vi "Nelder-Mead_alignment-max.vi"() -> (3 "Optimized Location":dbl[](array[numeric]), 10 "yStart":dbl=123.0 format="%#_13g", 11 "xStart":dbl=264.0 format="%#_13g")   [LabVIEW 2024]
uses:
  <vilib>/numeric/Random Number (Range) DBL.vi
  0b4b40c4-ef97-49a3-bff4-9c7e9883bc37.vi
  5b59031f-b1ff-41af-80a7-e72a33ebffa1.vi
  <vilib>/Array/Sort 2D Array - Pop Stack.vi
  <vilib>/Array/Sort 2D Array - Push Stack.vi
  0b4b40c4-ef97-49a3-bff4-9c7e9883bc37.vi/269d4b3b-47f5-49e3-8884-44851e4dd9d5.vi
  0b4b40c4-ef97-49a3-bff4-9c7e9883bc37.vi/6d99389c-673d-4efb-bf33-19b32bcf4cf8.vi
  5b59031f-b1ff-41af-80a7-e72a33ebffa1.vi/269d4b3b-47f5-49e3-8884-44851e4dd9d5.vi
  5b59031f-b1ff-41af-80a7-e72a33ebffa1.vi/6d99389c-673d-4efb-bf33-19b32bcf4cf8.vi
  <vilib>/Analysis/NI_AALBase.lvlib
panel:
  out "model-mode":bool
  out "elapsed time (s)":dbl
  out "n":i32(slide) scale=0.0..1000.0
  out "GrAsc - avgs":dbl[][](array[numeric])
  out "NM - avgs":dbl[][](array[numeric])
  in  "nTrials":i32=1000
  out "std dev of simplex values 2":dbl
  out "simplex leg lengths 2":dbl[](array[numeric])
  out "iterations timeout 2":bool
  out "simplex converge 2":bool
  out "value converge 2":bool
  out "Starting Points":dbl[][][](array[numeric])
  in  "k":dbl=50.0
  out "GrAsc res":dbl[](array[numeric])
  out "x_c":dbl[](array[numeric])
  out "x_e":dbl[](array[numeric])
  out "x_r":dbl[](array[numeric])
  out "x_o":dbl[](array[numeric])
  out "iterations timeout":bool
  out "simplex converge":bool
  out "value converge":bool
  out "simplex leg lengths":dbl[](array[numeric])
  out "std dev of simplex values":dbl
  in  "stop":bool
  # "Avg"
  # "Std Dev"
  # "X"
  # "Y"
  # "Value"
  # "n Trials"
  # "Failures"
  # "Avg"
  # "Std Dev"
  # "X"
  # "Y"
  # "Value"
  # "n Trials"
  # "Failures"
  # "centroid"
  # "reflection point"
  # "expansion point"
  # "contraction point"
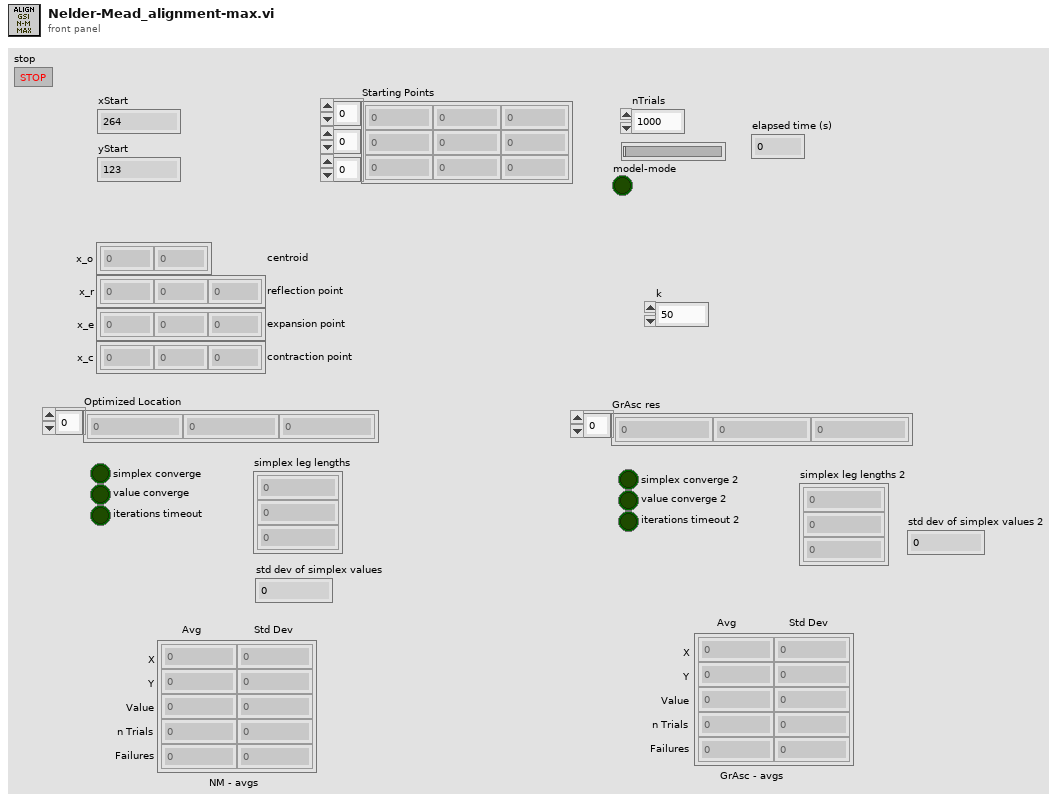
[diagram p1: front panel]
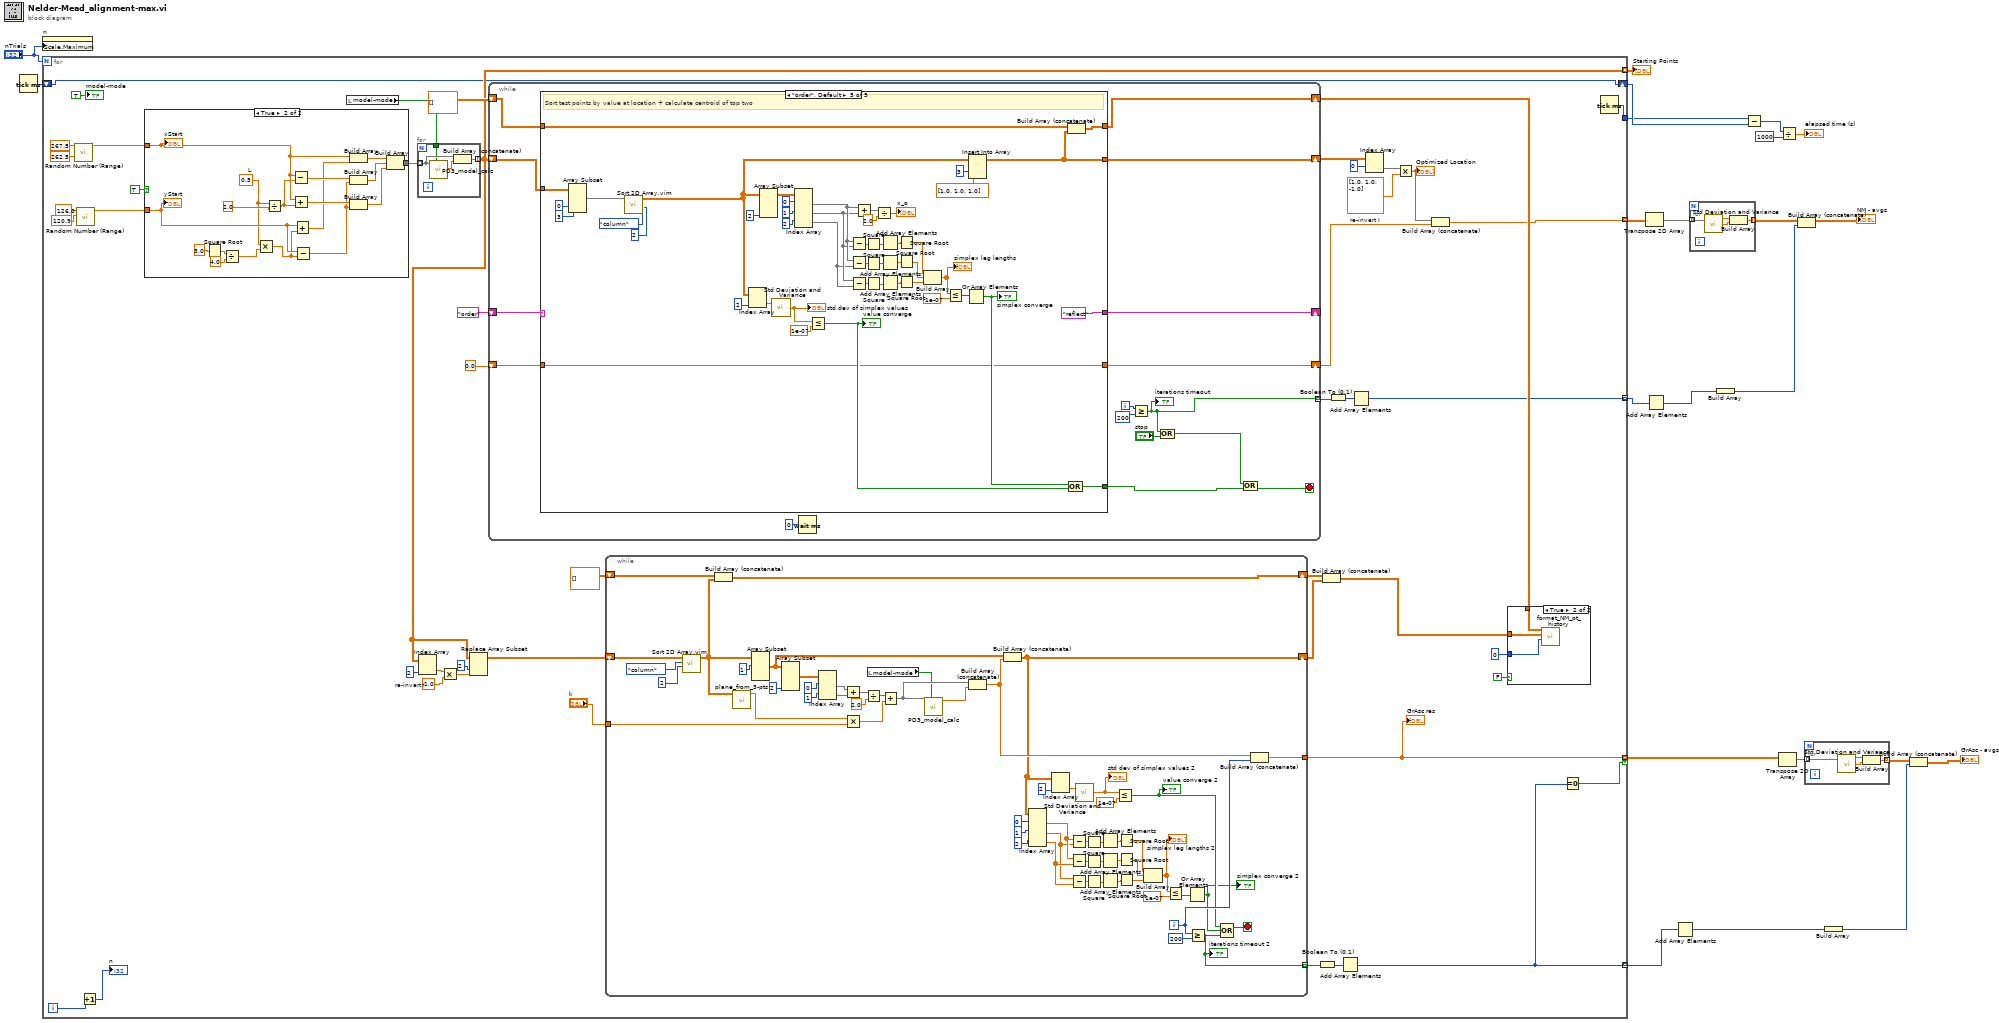
[diagram p0: block diagram]
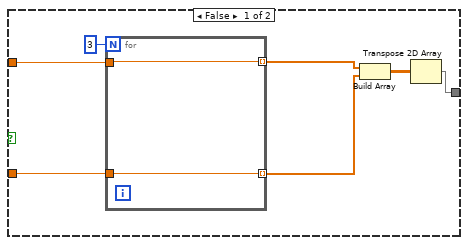
[diagram p3: hidden frame]
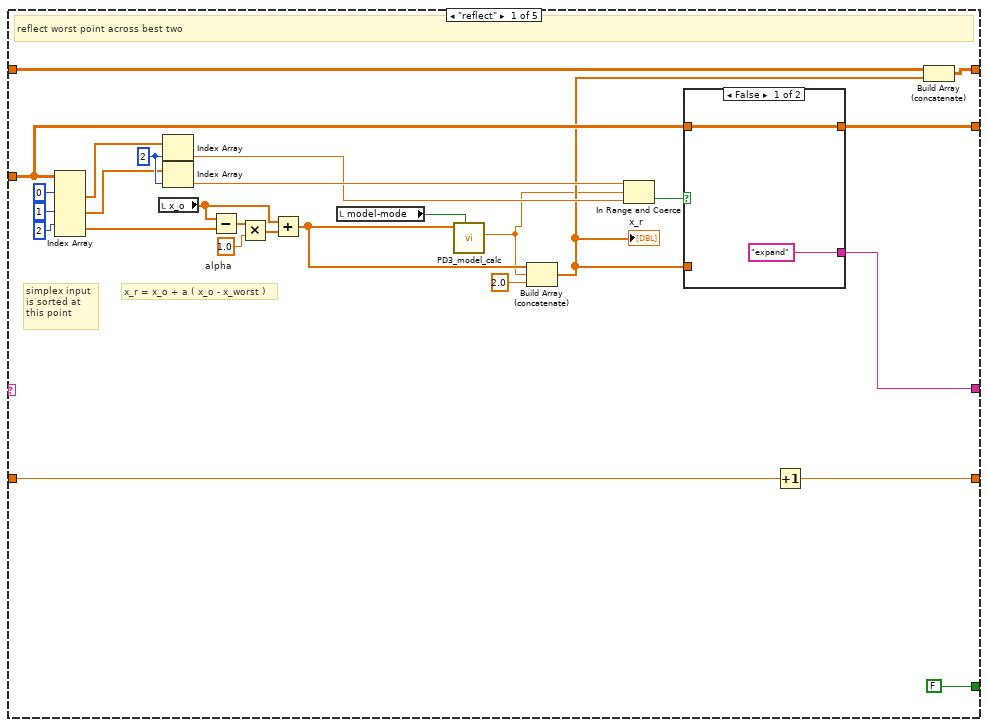
[diagram p4: hidden frame]
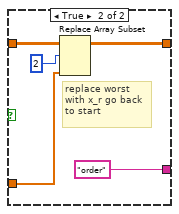
[diagram p5: hidden frame]
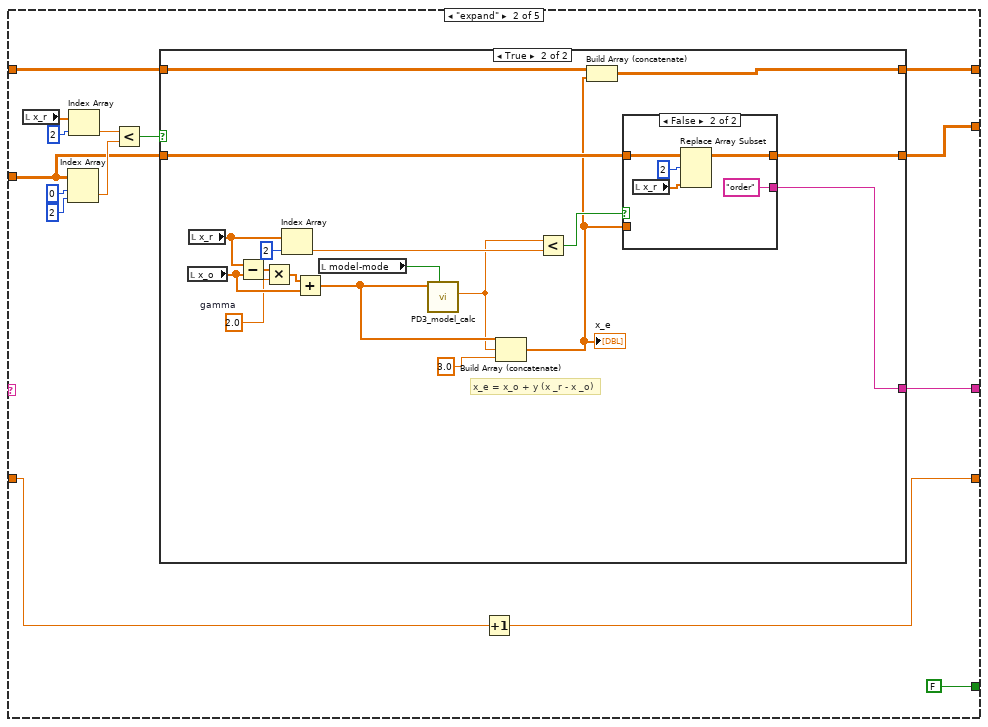
[diagram p6: hidden frame]
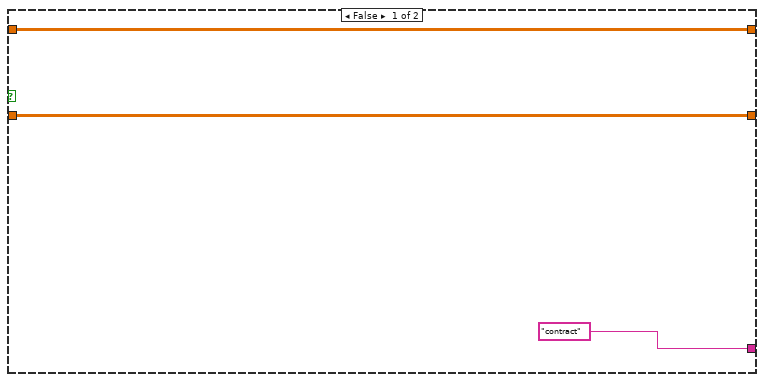
[diagram p7: hidden frame]
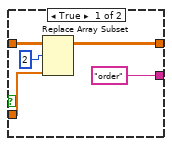
[diagram p8: hidden frame]
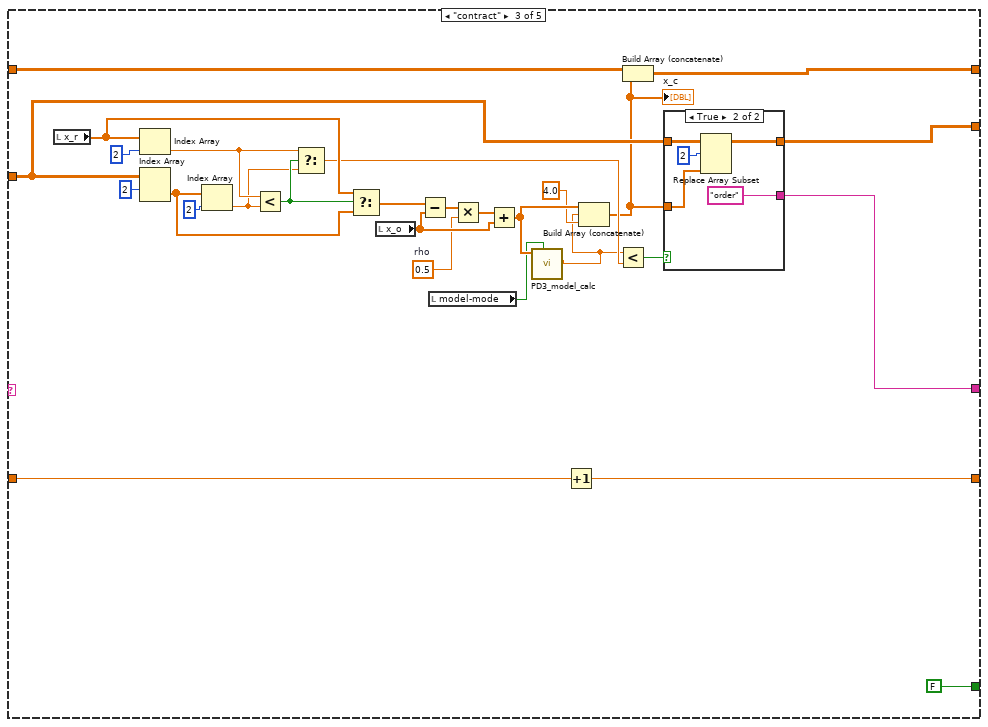
[diagram p9: hidden frame]
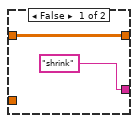
[diagram p10: hidden frame]
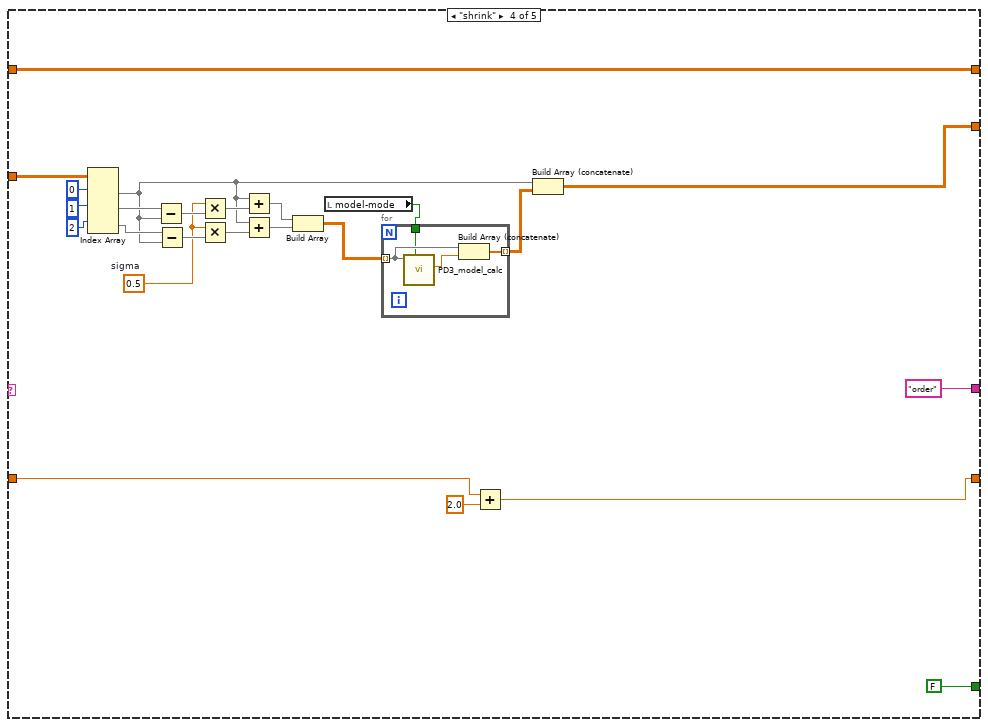
[diagram p11: hidden frame]
diagram:
  n1 = Tick Count (ms)() -> (millisecond timer value=w4:u32)
  n2 = property on="n" class="Slide (strict)"("Scale.Maximum"="nTrials") -> ()  [unwired: 2 in, 2 out]
  n3 = for {
    N: "nTrials" -> [_]
    tunnel: [w42] -> w21 mode=indexing
    tunnel: [w40] -> w20 mode=indexing
    tunnel: [w37] -> w15 mode=indexing if=w34
    tunnel: [w33] -> w14 mode=indexing
    tunnel: [w30] -> w10 mode=indexing
    shift-right: [w26] -> w3
    shift-left: w4 -> [w26]
    tunnel: [w25] -> w1
    i -> [w29]
    w57 = -1.0  # re-invert I
    w64 = dbl[] [1.0, 1.0, -1.0]  # re-invert I
    n4 = call-poly <vilib>:"Random Number (Range).vi"("lower bound (0)"=262.5, "upper bound (100)"=267.5) -> ("number"=w48:dbl)  [unwired: 9 in]
    n5 = call-poly <vilib>:"Random Number (Range).vi"("lower bound (0)"=120.9 ("upper bound (100)"), "upper bound (100)"=126.0 ("lower bound (0)")) -> ("number"=w47:dbl)  [unwired: 9 in]
    n6 = Increment(x=w29) -> (x+1=→"n":i32)
    n7 = case shown="True" TRUE {
      tunnel: [w73 w96] -> w52
      tunnel: w48 -> [w78 w88]
      tunnel: w47 -> [w77 w87]
      frame False {
        n8 = for {
          N: 3 -> [_]
          tunnel: w78 -> [w81]
          tunnel: [w81] -> w76 mode=indexing
          tunnel: w77 -> [w80]
          tunnel: [w80] -> w74 mode=indexing
        }
        n9 = Build Array(w76, w74) -> (w75:dbl[][])
        n10 = Transpose 2D Array(2D array=w75) -> (transposed array=w73:dbl[][])
      }
      frame True {
        w82 = 0.5  # L
        n11 = Square Root(x=3.0) -> (sqrt(x)=w95:dbl)
        n12 = Divide(x=w95, y=4.0) -> (x/y=w84:dbl)
        n13 = Multiply(x=w82, y=w84) -> (x*y=w83:dbl)
        n14 = Divide(x=w82, y=2.0) -> (x/y=w85:dbl)
        n15 = Subtract(x=w88, y=w85) -> (x-y=w92:dbl)
        n16 = Add(x=w88, y=w85) -> (x+y=w91:dbl)
        n17 = Add(x=w87, y=w83) -> (x+y=w90:dbl)
        n18 = Subtract(x=w87, y=w83) -> (x-y=w89:dbl)
        n19 = Build Array(w88, w90) -> (w97:dbl[])
        n20 = Build Array(w92, w89) -> (w98:dbl[])
        n21 = Build Array(w91, w89) -> (w99:dbl[])
        n22 = Build Array(w97, w98, w99) -> (w96:dbl[][])
        "xStart" <- w88
        "yStart" <- w87
      }
    }
    n23 = local read "model-mode"() -> (w23:bool)
    n24 = for {
      tunnel: w52 -> [w159] mode=indexing
      tunnel: [w160] -> w42 mode=indexing
      tunnel: w23 -> [w157]
      n25 = call "PD3_model_calc.vi"("mode"=w157, "pos_in"=w159) -> ("-I_out"=w158:dbl)  [unwired: 8 in, 1 out]
      n26 = Build Array (concatenate)(w159, w158) -> (w160:dbl[])
    }
    n27 = Index Array(array=w42, index (col)=2 ("disabled index (col)")) -> (element=w55:dbl[])  [unwired: 1 in]
    n28 = Multiply(x=w55, y=w57) -> (x*y=w53:dbl[])
    n29 = Replace Array Subset(array=w42, new element=w53, index (col)=2 ("disabled index (col)")) -> (w51:dbl[][])  [unwired: 1 in]
    n30 = while {
      shift-right: [w174] -> w69
      shift-left: w42 -> [w172]
      shift-right: [w175] -> _
      shift-left: "order" -> [w176]
      shift-right: [w170] -> w63
      shift-left: dbl[][] [] -> [w171]
      shift-right: [w164] -> w38
      shift-left: 0.0 -> [w165]
      tunnel: [w163] -> w31 mode=indexing
      i -> [w166]
      stop <- w162 stop-if-true
      n31 = case shown="\"order\", Default" w176 {
        tunnel: w172 -> [w188 w218 w270 w314 w358]
        tunnel: [FALSE FALSE FALSE FALSE w334] -> w168
        tunnel: [w187 w217 w271 w303 w323] -> w174
        tunnel: [w189 w216 w272 "order" "reflect"] -> w175
        tunnel: w171 -> [w185 w214 w266 w301 w322]
        tunnel: [w184 w213 w264 w301 w328] -> w170
        tunnel: w165 -> [w180 w212 w260 w295 w320]
        tunnel: [w179 w211 w259 w294 w320] -> w164
        frame "reflect" {
          w181 = 1.0  # alpha
          w197 = 2 ("index")
          # "simplex input\nis sorted at\nthis point"
          # "x_r = x_o + a ( x_o - x_worst )"
          # "reflect worst point across best two"
          n32 = Index Array(array=w188, index (row) #1=0 ("index (row)"), index (row) #2=1 ("index (row)"), index (row) #3=2 ("index (row)")) -> (element #1=w196:dbl[], element #2=w195:dbl[], element #3=w198:dbl[])  [unwired: 3 in]
          n33 = local read "x_o"() -> (w190:dbl[])
          n34 = Index Array(array=w196, index=w197) -> (element=w193:dbl)
          n35 = Index Array(array=w195, index=w197) -> (element=w194:dbl)
          n36 = Subtract(x=w190, y=w198) -> (x-y=w202:dbl[])
          n37 = Multiply(x=w202, y=w181) -> (x*y=w201:dbl[])
          n38 = Add(x=w190, y=w201) -> (x+y=w191:dbl[])
          n39 = local read "model-mode"() -> (w177:bool)
          n40 = call "PD3_model_calc.vi"("mode"=w177, "pos_in"=w191) -> ("-I_out"=w178:dbl)  [unwired: 8 in, 1 out]
          n41 = Build Array (concatenate)(w191, w178, 2.0) -> (w183:dbl[])
          "x_r" <- w183
          n42 = In Range and Coerce(upper limit=w194, x=w178, lower limit=w193) -> (In Range?=w192:bool)  [unwired: 1 out]
          n43 = case shown="False" w192 {
            tunnel: ["expand" "order"] -> w189
            tunnel: w188 -> [w204 w210]
            tunnel: [w204 w207] -> w187
            tunnel: w183 -> [_ w208]
            frame False {
            }
            frame True {
              # "replace worst \nwith x_r go back\nto start"
              n44 = Replace Array Subset(array=w210, new element=w208, index (row)=2) -> (w207:dbl[][])  [unwired: 1 in]
            }
          }
          n45 = Increment(x=w180) -> (x+1=w179:dbl)
          n46 = Build Array (concatenate)(w185, w183) -> (w184:dbl[][])
        }
        frame "expand" {
          n47 = local read "x_r"() -> (w223:dbl[])
          n48 = Index Array(array=w218, index (row)=0, index (col)=2 ("disabled index (col)")) -> (element=w221:dbl)
          n49 = Index Array(array=w223, index=2) -> (element=w220:dbl)
          n50 = Less?(x=w220, y=w221) -> (x < y?=w219:bool)
          n51 = case shown="True" w219 {
            tunnel: w218 -> [w228 w239]
            tunnel: [w228 w237] -> w217
            tunnel: ["contract" w236] -> w216
            tunnel: w214 -> [w226 w235]
            tunnel: [w226 w234] -> w213
            frame False {
            }
            frame True {
              w231 = 2.0  # gamma
              # "x_e = x_o + y (x _r - x _o)"
              n52 = local read "x_o"() -> (w244:dbl[])
              n53 = local read "x_r"() -> (w243:dbl[])
              n54 = Subtract(x=w243, y=w244) -> (x-y=w246:dbl[])
              n55 = Multiply(x=w246, y=w231) -> (x*y=w245:dbl[])
              n56 = Index Array(array=w243, index=2) -> (element=w241:dbl)
              n57 = Add(x=w245, y=w244) -> (x+y=w238:dbl[])
              n58 = local read "model-mode"() -> (w229:bool)
              n59 = call "PD3_model_calc.vi"("mode"=w229, "pos_in"=w238) -> ("-I_out"=w230:dbl)  [unwired: 8 in, 1 out]
              n60 = Build Array (concatenate)(w238, w230, 3.0) -> (w233:dbl[])
              "x_e" <- w233
              n61 = Less?(x=w230, y=w241) -> (x < y?=w240:bool)
              n62 = Build Array (concatenate)(w235, w233) -> (w234:dbl[][])
              n63 = case shown="False" w240 {
                tunnel: w239 -> [w250 w255]
                tunnel: w233 -> [w249 _]
                tunnel: [w248 w254] -> w237
                tunnel: ["order" "order"] -> w236
                frame True {
                  n64 = Replace Array Subset(array=w250, new element=w249, index (row)=2) -> (w248:dbl[][])  [unwired: 1 in]
                }
                frame False {
                  n65 = local read "x_r"() -> (w252:dbl[])
                  n66 = Replace Array Subset(array=w255, new element=w252, index (row)=2) -> (w254:dbl[][])  [unwired: 1 in]
                }
              }
            }
          }
          n67 = Increment(x=w212) -> (x+1=w211:dbl)
        }
        frame "contract" {
          w261 = 0.5  # rho
          n68 = local read "x_r"() -> (w281:dbl[])
          n69 = Index Array(array=w281, index=2) -> (element=w276:dbl)
          n70 = Index Array(array=w270, index (row)=2) -> (element=w280:dbl[])  [unwired: 1 in]
          n71 = Index Array(array=w280, index=2) -> (element=w275:dbl)
          n72 = Less?(x=w276, y=w275) -> (x < y?=w277:bool)
          n73 = Select(t=w276, s=w277, f=w275) -> (s? t:f=w274:dbl)
          n74 = Select(t=w281, s=w277, f=w280) -> (s? t:f=w279:dbl[])
          n75 = local read "x_o"() -> (w268:dbl[])
          n76 = Subtract(x=w279, y=w268) -> (x-y=w278:dbl[])
          n77 = local read "model-mode"() -> (w257:bool)
          n78 = Multiply(x=w278, y=w261) -> (x*y=w269:dbl[])
          n79 = Add(x=w269, y=w268) -> (x+y=w265:dbl[])
          n80 = call "PD3_model_calc.vi"("mode"=w257, "pos_in"=w265) -> ("-I_out"=w258:dbl)  [unwired: 8 in, 1 out]
          n81 = Increment(x=w260) -> (x+1=w259:dbl)
          n82 = Build Array (concatenate)(w265, w258, 4.0 ("array")) -> (w263:dbl[])
          "x_c" <- w263
          n83 = Less?(x=w258, y=w274) -> (x < y?=w273:bool)
          n84 = Build Array (concatenate)(w266, w263) -> (w264:dbl[][])
          n85 = case shown="True" w273 {
            tunnel: ["shrink" "order"] -> w272
            tunnel: [w285 w287] -> w271
            tunnel: w270 -> [w285 w289]
            tunnel: w263 -> [_ w288]
            frame False {
            }
            frame True {
              n86 = Replace Array Subset(array=w289, new element=w288, index (row)=2) -> (w287:dbl[][])  [unwired: 1 in]
            }
          }
        }
        frame "shrink" {
          w300 = 0.5  # sigma
          n87 = Index Array(array=w314, index (row) #1=0 ("index (row)"), index (row) #2=1 ("index (row)"), index (row) #3=2 ("index (row)")) -> (element #1=w304:dbl[], element #2=w310:dbl[], element #3=w309:dbl[])  [unwired: 3 in]
          n88 = Subtract(x=w310, y=w304) -> (x-y=w307:dbl[])
          n89 = Subtract(x=w309, y=w304) -> (x-y=w308:dbl[])
          n90 = Multiply(x=w300, y=w307) -> (x*y=w306:dbl[])
          n91 = Multiply(x=w300, y=w308) -> (x*y=w305:dbl[])
          n92 = Add(x=w304, y=w306) -> (x+y=w299:dbl[])
          n93 = Add(x=w304, y=w305) -> (x+y=w298:dbl[])
          n94 = Build Array(w299, w298) -> (w297:dbl[][])
          n95 = local read "model-mode"() -> (w292:bool)
          n96 = for {
            tunnel: w297 -> [w318] mode=indexing
            tunnel: [w319] -> w296 mode=indexing
            tunnel: w292 -> [w316]
            n97 = call "PD3_model_calc.vi"("mode"=w316, "pos_in"=w318) -> ("-I_out"=w317:dbl)  [unwired: 8 in, 1 out]
            n98 = Build Array (concatenate)(w318, w317) -> (w319:dbl[])
          }
          n99 = Add(x=w295, y=2.0) -> (x+y=w294:dbl)
          n100 = Build Array (concatenate)(w304, w296) -> (w303:dbl[][])
        }
        frame "order", Default {
          # "Sort test points by value at location + calculate centroid of top two"
          n101 = Array Subset(array=w358, index (col)=0 ("index"), length (col)=3 ("length")) -> (w321:dbl[][])  [unwired: 2 in]
          n102 = call "Sort 2D Array.vim"("index"=2, "dimension to index (column)"=enum16{"column", "row"}."column", "2D array"=w321) -> ("sorted 2D array"=w326:dbl[][])  [unwired: 7 in, 1 out]
          n103 = Index Array(array=w326, index (col)=2 ("index")) -> (element=w352:dbl[])  [unwired: 1 in]
          n104 = Array Subset(array=w326, length (col)=2 ("length")) -> (w351:dbl[][])  [unwired: 3 in]
          n105 = call <vilib>:"Std Deviation and Variance.vi"("X"=w352) -> ("standard deviation"=w327:dbl)  [unwired: 1 in, 2 out]
          "std dev of simplex values" <- w327
          n106 = Index Array(array=w351, index (row) #1=0 ("index (row)"), index (row) #2=1 ("index (row)"), index (row) #3=2 ("index (row)")) -> (element #1=w331:dbl[], element #2=w330:dbl[], element #3=w329:dbl[])  [unwired: 3 in]
          n107 = Less Or Equal?(x=w327, y=1e-07) -> (x <= y?=w333:bool)
          "value converge" <- w333
          n108 = Subtract(x=w331, y=w330) -> (x-y=w349:dbl[])
          n109 = Subtract(x=w331, y=w329) -> (x-y=w341:dbl[])
          n110 = Subtract(x=w330, y=w329) -> (x-y=w344:dbl[])
          n111 = Add(x=w331, y=w330) -> (x+y=w356:dbl[])
          n112 = Square(x=w349) -> (x^2=w348:dbl[])
          n113 = Square(x=w341) -> (x^2=w345:dbl[])
          n114 = Square(x=w344) -> (x^2=w343:dbl[])
          n115 = Divide(x=w356, y=2.0) -> (x/y=→"x_o":dbl[])
          n116 = Add Array Elements(numeric array=w348) -> (sum=w347:dbl)
          n117 = Add Array Elements(numeric array=w345) -> (sum=w346:dbl)
          n118 = Add Array Elements(numeric array=w343) -> (sum=w342:dbl)
          n119 = Square Root(x=w347) -> (sqrt(x)=w338:dbl)
          n120 = Square Root(x=w346) -> (sqrt(x)=w339:dbl)
          n121 = Square Root(x=w342) -> (sqrt(x)=w340:dbl)
          n122 = Build Array(w338, w339, w340) -> (w337:dbl[])
          "simplex leg lengths" <- w337
          n123 = Less Or Equal?(x=w337, y=1e-07) -> (x <= y?=w335:bool[])
          n124 = Or Array Elements(Boolean array=w335) -> (logical OR=w332:bool)
          "simplex converge" <- w332
          n125 = Insert Into Array(array=w326, index (col)=3 ("disabled index (col)"), new element=dbl[] [1.0, 1.0, 1.0] ("new element/subarray")) -> (w323:dbl[][])  [unwired: 1 in]
          n126 = Build Array (concatenate)(w322, w323) -> (w328:dbl[][])
          n127 = Compound Arithmetic op=OR(w332, w333) -> (w334:bool)
        }
      }
      n128 = Wait (ms)(milliseconds to wait=u32 0) -> ()  [unwired: 1 out]
      n129 = Greater Or Equal?(x=w166, y=200) -> (x >= y?=w163:bool)
      "iterations timeout" <- w163
      n130 = Compound Arithmetic op=OR(w163, "stop") -> (w161:bool)
      n131 = Compound Arithmetic op=OR(w161, w168) -> (w162:bool)
    }
    n132 = while {
      tunnel: "k" -> [w134]
      shift-right: [w137] -> w50
      shift-left: dbl[][] [] -> [w156]
      shift-right: [w115] -> w49
      shift-left: w51 -> [w153]
      tunnel: [w129] -> w37
      tunnel: [w102] -> w36 mode=indexing
      i -> [w128]
      stop <- w130 stop-if-true
      n133 = call "Sort 2D Array.vim"("index"=2, "dimension to index (column)"=enum16{"column", "row"}."column", "2D array"=w153) -> ("sorted 2D array"=w136:dbl[][])  [unwired: 7 in, 1 out]
      n134 = Build Array (concatenate)(w156, w136) -> (w137:dbl[][])
      n135 = call "plane_from_3-pts.vi"("Input"=w136) -> ("gradient-out"=w139:dbl[])  [unwired: 9 in, 1 out]
      n136 = Array Subset(array=w136, index (row)=1 ("index")) -> (w143:dbl[][])  [unwired: 3 in]
      n137 = Array Subset(array=w143, length (col)=2 ("length")) -> (w144:dbl[][])  [unwired: 3 in]
      n138 = Index Array(array=w144, index (row) #1=0 ("index (row)"), index (row) #2=1 ("index (row)")) -> (element #1=w149:dbl[], element #2=w148:dbl[])  [unwired: 2 in]
      n139 = Add(x=w149, y=w148) -> (x+y=w147:dbl[])
      n140 = Multiply(x=w139, y=w134) -> (x*y=w140:dbl[])
      n141 = Divide(x=w147, y=2.0) -> (x/y=w142:dbl[])
      n142 = local read "model-mode"() -> (w100:bool)
      n143 = Add(x=w142, y=w140) -> (x+y=w141:dbl[])
      n144 = call "PD3_model_calc.vi"("mode"=w100, "pos_in"=w141) -> ("+I_out"=w101:dbl)  [unwired: 8 in, 1 out]
      n145 = Build Array (concatenate)(w141, w101) -> (w135:dbl[])
      n146 = Build Array (concatenate)(w143, w135) -> (w115:dbl[][])
      n147 = Index Array(array=w115, index (row) #1=0 ("index (row)"), index (row) #2=1 ("index (row)"), index (row) #3=2 ("index (row)")) -> (element #1=w114:dbl[], element #2=w112:dbl[], element #3=w113:dbl[])  [unwired: 3 in]
      n148 = Index Array(array=w115, index (col)=2 ("index")) -> (element=w133:dbl[])  [unwired: 1 in]
      n149 = Subtract(x=w114, y=w112) -> (x-y=w116:dbl[])
      n150 = Subtract(x=w114, y=w113) -> (x-y=w124:dbl[])
      n151 = Subtract(x=w112, y=w113) -> (x-y=w121:dbl[])
      n152 = call <vilib>:"Std Deviation and Variance.vi"("X"=w133) -> ("standard deviation"=w103:dbl)  [unwired: 1 in, 2 out]
      "std dev of simplex values 2" <- w103
      n153 = Square(x=w116) -> (x^2=w117:dbl[])
      n154 = Square(x=w124) -> (x^2=w120:dbl[])
      n155 = Square(x=w121) -> (x^2=w122:dbl[])
      n156 = Add Array Elements(numeric array=w117) -> (sum=w118:dbl)
      n157 = Add Array Elements(numeric array=w120) -> (sum=w119:dbl)
      n158 = Add Array Elements(numeric array=w122) -> (sum=w123:dbl)
      n159 = Less Or Equal?(x=w103, y=1e-07) -> (x <= y?=w106:bool)
      "value converge 2" <- w106
      n160 = Square Root(x=w118) -> (sqrt(x)=w127:dbl)
      n161 = Square Root(x=w119) -> (sqrt(x)=w126:dbl)
      n162 = Square Root(x=w123) -> (sqrt(x)=w125:dbl)
      n163 = Build Array(w127, w126, w125) -> (w104:dbl[])
      "simplex leg lengths 2" <- w104
      n164 = Less Or Equal?(x=w104, y=1e-07) -> (x <= y?=w110:bool[])
      n165 = Or Array Elements(Boolean array=w110) -> (logical OR=w105:bool)
      "simplex converge 2" <- w105
      n166 = Greater Or Equal?(x=w128, y=200) -> (x >= y?=w102:bool)
      "iterations timeout 2" <- w102
      n167 = Compound Arithmetic op=OR(w106, w105, w102) -> (w130:bool)
      n168 = Build Array (concatenate)(w135, w128) -> (w129:dbl[])
    }
    "GrAsc res" <- w37
    n169 = Boolean To (0,1)(Boolean=w36) -> (0, 1=w35:i16[])
    n170 = Build Array (concatenate)(w50, w49) -> (w45:dbl[][])
    n171 = Boolean To (0,1)(Boolean=w31) -> (0, 1=w32:i16[])
    n172 = Add Array Elements(numeric array=w35) -> (sum=w33:i16)
    n173 = Add Array Elements(numeric array=w32) -> (sum=w30:i16)
    n174 = Index Array(array=w69, index (row)=0) -> (element=w65:dbl[])  [unwired: 1 in]
    n175 = Multiply(x=w65, y=w64) -> (x*y=w41:dbl[])
    "Optimized Location" <- w41
    n176 = Build Array (concatenate)(w41, w38) -> (w40:dbl[])
    n177 = case shown="True" FALSE {
      tunnel: w63 -> [_ w72]
      tunnel: w45 -> [_ w71]
      tunnel: 0 ("trial #") -> [_ w70]
      frame False {
      }
      frame True {
        n178 = call "format_NM_pt_history.vi"("trial #"=w70, "GrAsc in"=w71, "NM in"=w72) -> ()  [unwired: 9 in]
      }
    }
    n179 = Equal To 0?(x=w33) -> (x = 0?=w34:bool)
    n180 = Tick Count (ms)() -> (millisecond timer value=w25:u32)
    "model-mode" <- TRUE
  }
  "Starting Points" <- w21
  n181 = Transpose 2D Array(2D array=w20) -> (transposed array=w19:dbl[][])
  n182 = Add Array Elements(numeric array=w10) -> (sum=w11:i16)
  n183 = Add Array Elements(numeric array=w14) -> (sum=w13:i16)
  n184 = for {
    tunnel: w19 -> [w370] mode=indexing
    tunnel: [w367] -> w18 mode=indexing
    n185 = call <vilib>:"Std Deviation and Variance.vi"("X"=w370) -> ("mean"=w369:dbl, "standard deviation"=w368:dbl)  [unwired: 1 in, 1 out]
    n186 = Build Array(w369, w368) -> (w367:dbl[])
  }
  n187 = Build Array(w11) -> (w8:i16[])
  n188 = Subtract(x=w1, y=w3) -> (x-y=w6:u32)
  n189 = Transpose 2D Array(2D array=w15) -> (transposed array=w16:dbl[][])
  n190 = Divide(x=w6, y=u32 1000) -> (x/y=→"elapsed time (s)":dbl)
  n191 = Build Array (concatenate)(w18, w8) -> (→"NM - avgs":dbl[][])
  n192 = for {
    tunnel: w16 -> [w371] mode=indexing
    tunnel: [w372] -> w17 mode=indexing
    n193 = call <vilib>:"Std Deviation and Variance.vi"("X"=w371) -> ("mean"=w374:dbl, "standard deviation"=w373:dbl)  [unwired: 1 in, 1 out]
    n194 = Build Array(w374, w373) -> (w372:dbl[])
  }
  n195 = Build Array(w13) -> (w12:i16[])
  n196 = Build Array (concatenate)(w17, w12) -> (→"GrAsc - avgs":dbl[][])
